vi "CmdExe.StdErr and Rtn Code to Error.vi"(5 "StdErr":string, 7 "RtnCode":i32, 10 "error in":errorcluster, 11 "App":string) -> (2 "error out":errorcluster)   [LabVIEW 2018]
uses:
  Errors/Error.Error Code List.ctl
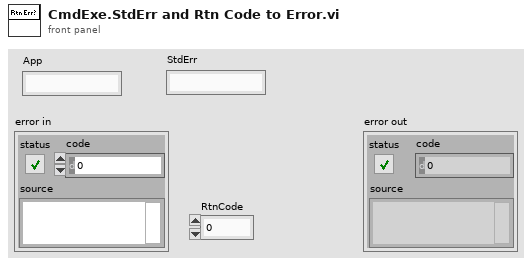
[diagram p1: front panel]
types:
  T1 = typedef "Error.Error Code List.ctl" = i32
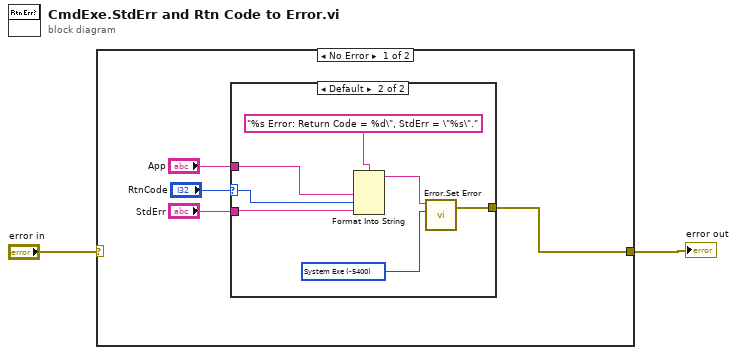
[diagram p0: block diagram]
diagram:
  n1 = case shown="No Error" "error in" {
    selector: "error in" -> [_ w14]
    tunnel: [w3 w14] -> w1
    frame No Error {
      n2 = case shown="Default" "RtnCode" {
        selector: "RtnCode" -> [_ w11]
        tunnel: "StdErr" -> [_ w12]
        tunnel: "App" -> [_ w10]
        tunnel: [_ w7] -> w3
        frame 0 {
        }
        frame Default {
          w8 = T1 -5400 items=["No Error"=0, "Abort"=-2, "Misc"=-5000, "Fixture Error"=-5100, "File IO - General"=-5200, "FIle IO - Config Error"=-5201, "Instrument - General"=-5300, "Instrument - Serial Com"=-5301, "Instrument - Camera"=-5302, "Instrument - PS"=-5303, "Instrument - Oscilloscope"=-5304, "Instrument - Function Gen"=-5305, "Instrument - Load"=-5306, "Instrument - Meter"=-5307, "Instrument - Power Control"=-5308, "Instrument - Motion"=-5309, "Instrument - RF"=-5310, "System Exe"=-5400, "Image Processing"=-5500, "Communication"=-5600, "Script - Syntax Error"=-6000, "Script - Invalid Name or Param"=-6100, "Script - Timeout"=-6200, "Invalid Data"=-6300, "FW Update Error"=-6500] ("Std Code")
          n3 = Format Into String(format string="%s Error: Return Code = %d\", StdErr = \"%s\".", w10, w11, w12) -> (resulting string=w9:string)  [unwired: 2 in, 1 out]
          n4 = call "Error.Set Error.vi"("Code"=w8, "Desc"=w9) -> ("error out"=w7:errorcluster)  [unwired: 5 in]
        }
      }
    }
    frame Error {
    }
  }
  "error out" <- w1
